vi "Bold Description String.vi"(8 "error in (no error)":errorcluster, 9 "Selection":T1, 10 "String":string, 11 "String Ref":refnum<vi>) -> (0 "error out":errorcluster)   [LabVIEW 2023, in "VI Properties Editor.lvlib"]
doc: "Bolds a string with bold tags in it, modifying the selection to keep it the same as before."
uses:
  VI Properties Editor.lvlib
  <vilib>/Utility/miscctls.llb/LVSelectionTypeDef.ctl
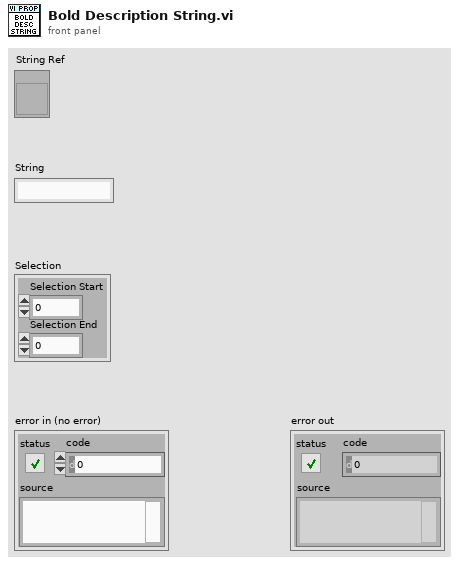
[diagram p1: front panel]
types:
  T1 = typedef "LVSelectionTypeDef.ctl" = cluster{"Selection Start":u32, "Selection End":u32}
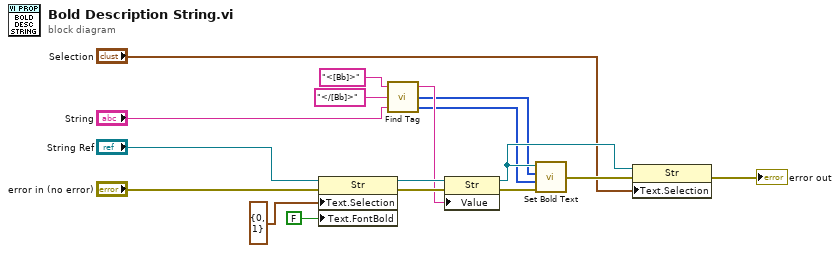
[diagram p0: block diagram]
diagram:
  n1 = property class="Str"(reference="String Ref", error in="error in (no error)", "Text.Selection"=T1 {"Selection Start"=0, "Selection End"=1}, "Text.FontBold"=FALSE ("Text.Font:Bold")) -> (reference out=w8:refnum<vi>, error out=w13:errorcluster)
  n2 = call <vilib>:"Find Tag.vi"("string"="String", "close tag"="</[Bb]>", "open tag"="<[Bb]>") -> ("Length"=w3:i32[], "Start"=w4:i32[], "string out"=w5:string)
  n3 = property class="Str"(reference=w8, error in=w13, "Value"=w5) -> (reference out=w10:refnum<vi>, error out=w14:errorcluster)
  n4 = call <vilib>:"Set Bold Text.vi"("error in"=w14, "Length"=w3, "Start"=w4, "text"=w10) -> ("error out"=w15:errorcluster)  [unwired: 2 in]
  n5 = property class="Str"(reference=w10, error in=w15, "Text.Selection"="Selection") -> (error out=→"error out":errorcluster)  [unwired: 1 out]
